vi "reward_behavior_michelle_visjitter.vi"() -> ()   [LabVIEW 2019]
doc: "The myRIO Project template acquires acceleration data from the onboard accelerometer and displays the changes of acceleration values in a waveform chart."
uses:
  <vilib>/myRIO/Common/Instrument Driver Framework/Utilities/typedefs/Generic FPGA Reference.ctl
  <vilib>/myRIO/Common/Instrument Driver Framework/Utilities/typedefs/myRIO v1.0 Reference.ctl
  <vilib>/myRIO/Common/Instrument Driver Framework/Utilities/typedefs/Hardware Version Enum.ctl
  <vilib>/myRIO/Common/Instrument Driver Framework/Utilities/typedefs/myRIO Generic Hardware Reference.ctl
  <vilib>/userdefined/High Color/nirio_resource_hc.ctl
  <vilib>/myRIO/Common/Instrument Driver Framework/Utilities/vis/Is FPGA Ref Available.vi
  <vilib>/myRIO/Common/Instrument Driver Framework/myRIO v1.0/Encoder/typedefs/Encoder Signal Mode.ctl
  <vilib>/myRIO/Common/Instrument Driver Framework/myRIO v1.0/Encoder/typedefs/Encoder Channels Enum.ctl
  <vilib>/myRIO/Instrument Drivers/Onboard IO/Encoder/typedefs/Encoder Reference.ctl
  <vilib>/myRIO/Instrument Drivers/Onboard IO/Encoder/Encoder.lvlib
  <vilib>/myRIO/Instrument Drivers/Onboard IO/Encoder/vis/Read.vi
  <vilib>/myRIO/Common/Instrument Driver Framework/myRIO v1.0/Encoder/typedefs/Encoder Configuration v1.0.ctl
  <vilib>/myRIO/Common/Instrument Driver Framework/myRIO v1.0/Encoder/vis/myRIO v1.1 Open Encoder.vi
  <vilib>/myRIO/Common/Instrument Driver Framework/myRIO v1.0/Encoder/vis/myRIO v1.0 Configure Encoder.vi
  <vilib>/myRIO/Instrument Drivers/Onboard IO/Encoder/vis/myRIO Encoder Open.xnode
  <vilib>/myRIO/Express VI/Onboard IO/Encoder/Encoder Express VI.xnode
  <vilib>/myRIO/Express VI/Onboard IO/DI/DI Express VI.xnode
  <vilib>/myRIO/Instrument Drivers/Onboard IO/DIO/vis/Read.vi
  <vilib>/myRIO/Instrument Drivers/Onboard IO/DIO/DIO.lvlib
  <vilib>/myRIO/Common/Instrument Driver Framework/myRIO v1.0/DIO/typedefs/DIO Channels Enum.ctl
  <vilib>/myRIO/Common/Instrument Driver Framework/myRIO v1.0/DIO/typedefs/DIO Channels List.ctl
  <vilib>/myRIO/Instrument Drivers/Onboard IO/DIO/typedefs/DIO Reference.ctl
  <vilib>/myRIO/Instrument Drivers/Onboard IO/DIO/vis/myRIO DIO Open.xnode
  <vilib>/myRIO/Common/Instrument Driver Framework/myRIO v1.0/DIO/vis/myRIO v1.1 Open DIO.vi
  <vilib>/myRIO/Instrument Drivers/Onboard IO/DIO/vis/Write.vi
  <vilib>/myRIO/Express VI/Onboard IO/DO/DO Express VI.xnode
  <vilib>/Analysis/Matrix/Datatypes/RealMatrix.ctl
  <vilib>/Analysis/Matrix/NI_Matrix.lvlib
panel:
  in  "Give reward":bool
  out "Timings":dbl[](array[numeric])
  out "ISI":dbl
  out "ISI start time":dbl
  out "Time_out":bool=TRUE
  out "Time since lick":dbl
  out "Time of last lick":dbl
  out "Rewarded trials":dbl[](array[numeric])
  out "Rewards":u16
  out "Active Trial":bool
  out "Array temp2":T1
  out "Stimuli Loaded":bool
  out "Stim_ID":dbl[](array[numeric])
  out "Reward_mat":dbl[](array[numeric])
  out "Reward":bool=TRUE
  out "Frame clock":i32
  out "Licks":u32
  out "Lick":bool
  out "Time":dbl
  out "Stop":bool
  in  "Frames to collect":u32
  out "Overflow?":bool
  out "Counter Value":i32
  out "Velocity":dbl
  out "Velocity Plot":dbl[](graph)
  out "Velocity array":dbl[](array[numeric])
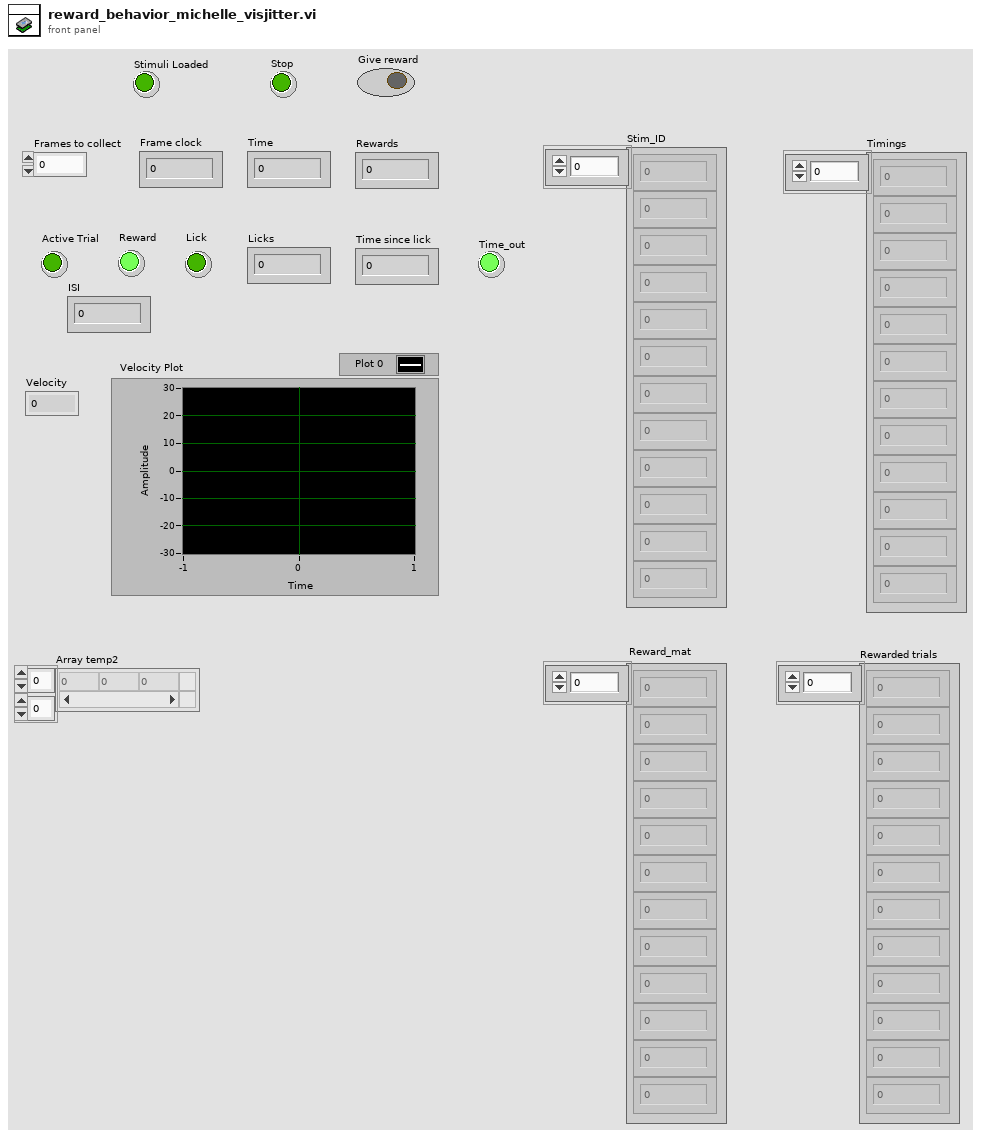
[diagram p1: front panel]
types:
  T1 = typedef "NI_Matrix.lvlib/RealMatrix.ctl" = dbl[][]
  T2 = typedef "Encoder.lvlib/Encoder Reference.ctl" = cluster{"myRIO Reference":T3, "Encoder Channels Enum":T7}
  T3 = typedef "myRIO Generic Hardware Reference.ctl" = cluster{"myRIO Model":T4, "myRIO Hardware Reference":T5}
  T4 = typedef "Hardware Version Enum.ctl" = enum16{"Unknown", "myRIO-1900", "myRIO-1950", "roboRIO", "NI ELVIS RIO CM", "ELVIS III"}
  T5 = typedef "myRIO v1.0 Reference.ctl" = cluster{"Generic FPGA Reference":T6, "Allow multiple opens":bool}
  T6 = typedef "Generic FPGA Reference.ctl" = refnum<k20>
  T7 = typedef "Encoder Channels Enum.ctl" = enum16{"Not Connected", "C/ENC0", "C/ENC1", "A/ENC", "A/ENC0", "A/ENC1", "A/ENC2", "A/ENC3", "A/ENC4", "A/ENC5", "A/ENC6", "A/ENC7", "A/ENC8", "A/ENC9", "B/ENC", "B/ENC0", "B/ENC1", "B/ENC2", "B/ENC3", "B/ENC4", "B/ENC5", "B/ENC6", "B/ENC7", "B/ENC8", "B/ENC9", "DIO/ENC0", "DIO/ENC1", "DIO/ENC2", "DIO/ENC3", "DIO/ENC4"}
  T8 = typedef "Encoder Signal Mode.ctl" = enum16{"Quadrature phase signal", "Step and direction signal"}
  T9 = typedef "nirio_resource_hc.ctl" = tag
  T10 = typedef "DIO.lvlib/DIO Reference.ctl" = cluster{"myRIO Reference":T3, "DIO Channels List":T11}
  T11 = typedef "DIO Channels List.ctl" = T12[]
  T12 = typedef "DIO Channels Enum.ctl" = enum16{"Not Connected", "C/DIO0", "C/DIO1", "C/DIO2", "C/DIO3", "C/DIO4", "C/DIO5", "C/DIO6", "C/DIO7", "A/DIO0", "A/DIO1", "A/DIO2", "A/DIO3", "A/DIO4", "A/DIO5", "A/DIO6", "A/DIO7", "A/DIO8", "A/DIO9", "A/DIO10", "A/DIO11", "A/DIO12", "A/DIO13", "A/DIO14", "A/DIO15", "A/DIO16", "A/DIO17", "A/DIO18", "A/DIO19", "B/DIO0", "B/DIO1", "B/DIO2", "B/DIO3", "B/DIO4", "B/DIO5", "B/DIO6", "B/DIO7", "B/DIO8", "B/DIO9", "B/DIO10", "B/DIO11", "B/DIO12", "B/DIO13", "B/DIO14", "B/DIO15", "B/DIO16", "B/DIO17", "B/DIO18", "B/DIO19", "LED0", "LED1", "LED2", "LED3", "Button0", "DIO/DIO0", "DIO/DIO1", "DIO/DIO2", "DIO/DIO3", "DIO/DIO4", "DIO/DIO5", "DIO/DIO6", "DIO/DIO7", "DIO/DIO8", "DIO/DIO9", "SPI/CS0", "SPI/CS1", "SPI/CS2", "SPI/CS3", "LED RADIO (Green)", "LED RADIO (Red)", "LED COMM (Green)", "LED COMM (Red)", "LED MODE (Green)", "LED MODE (Red)"}
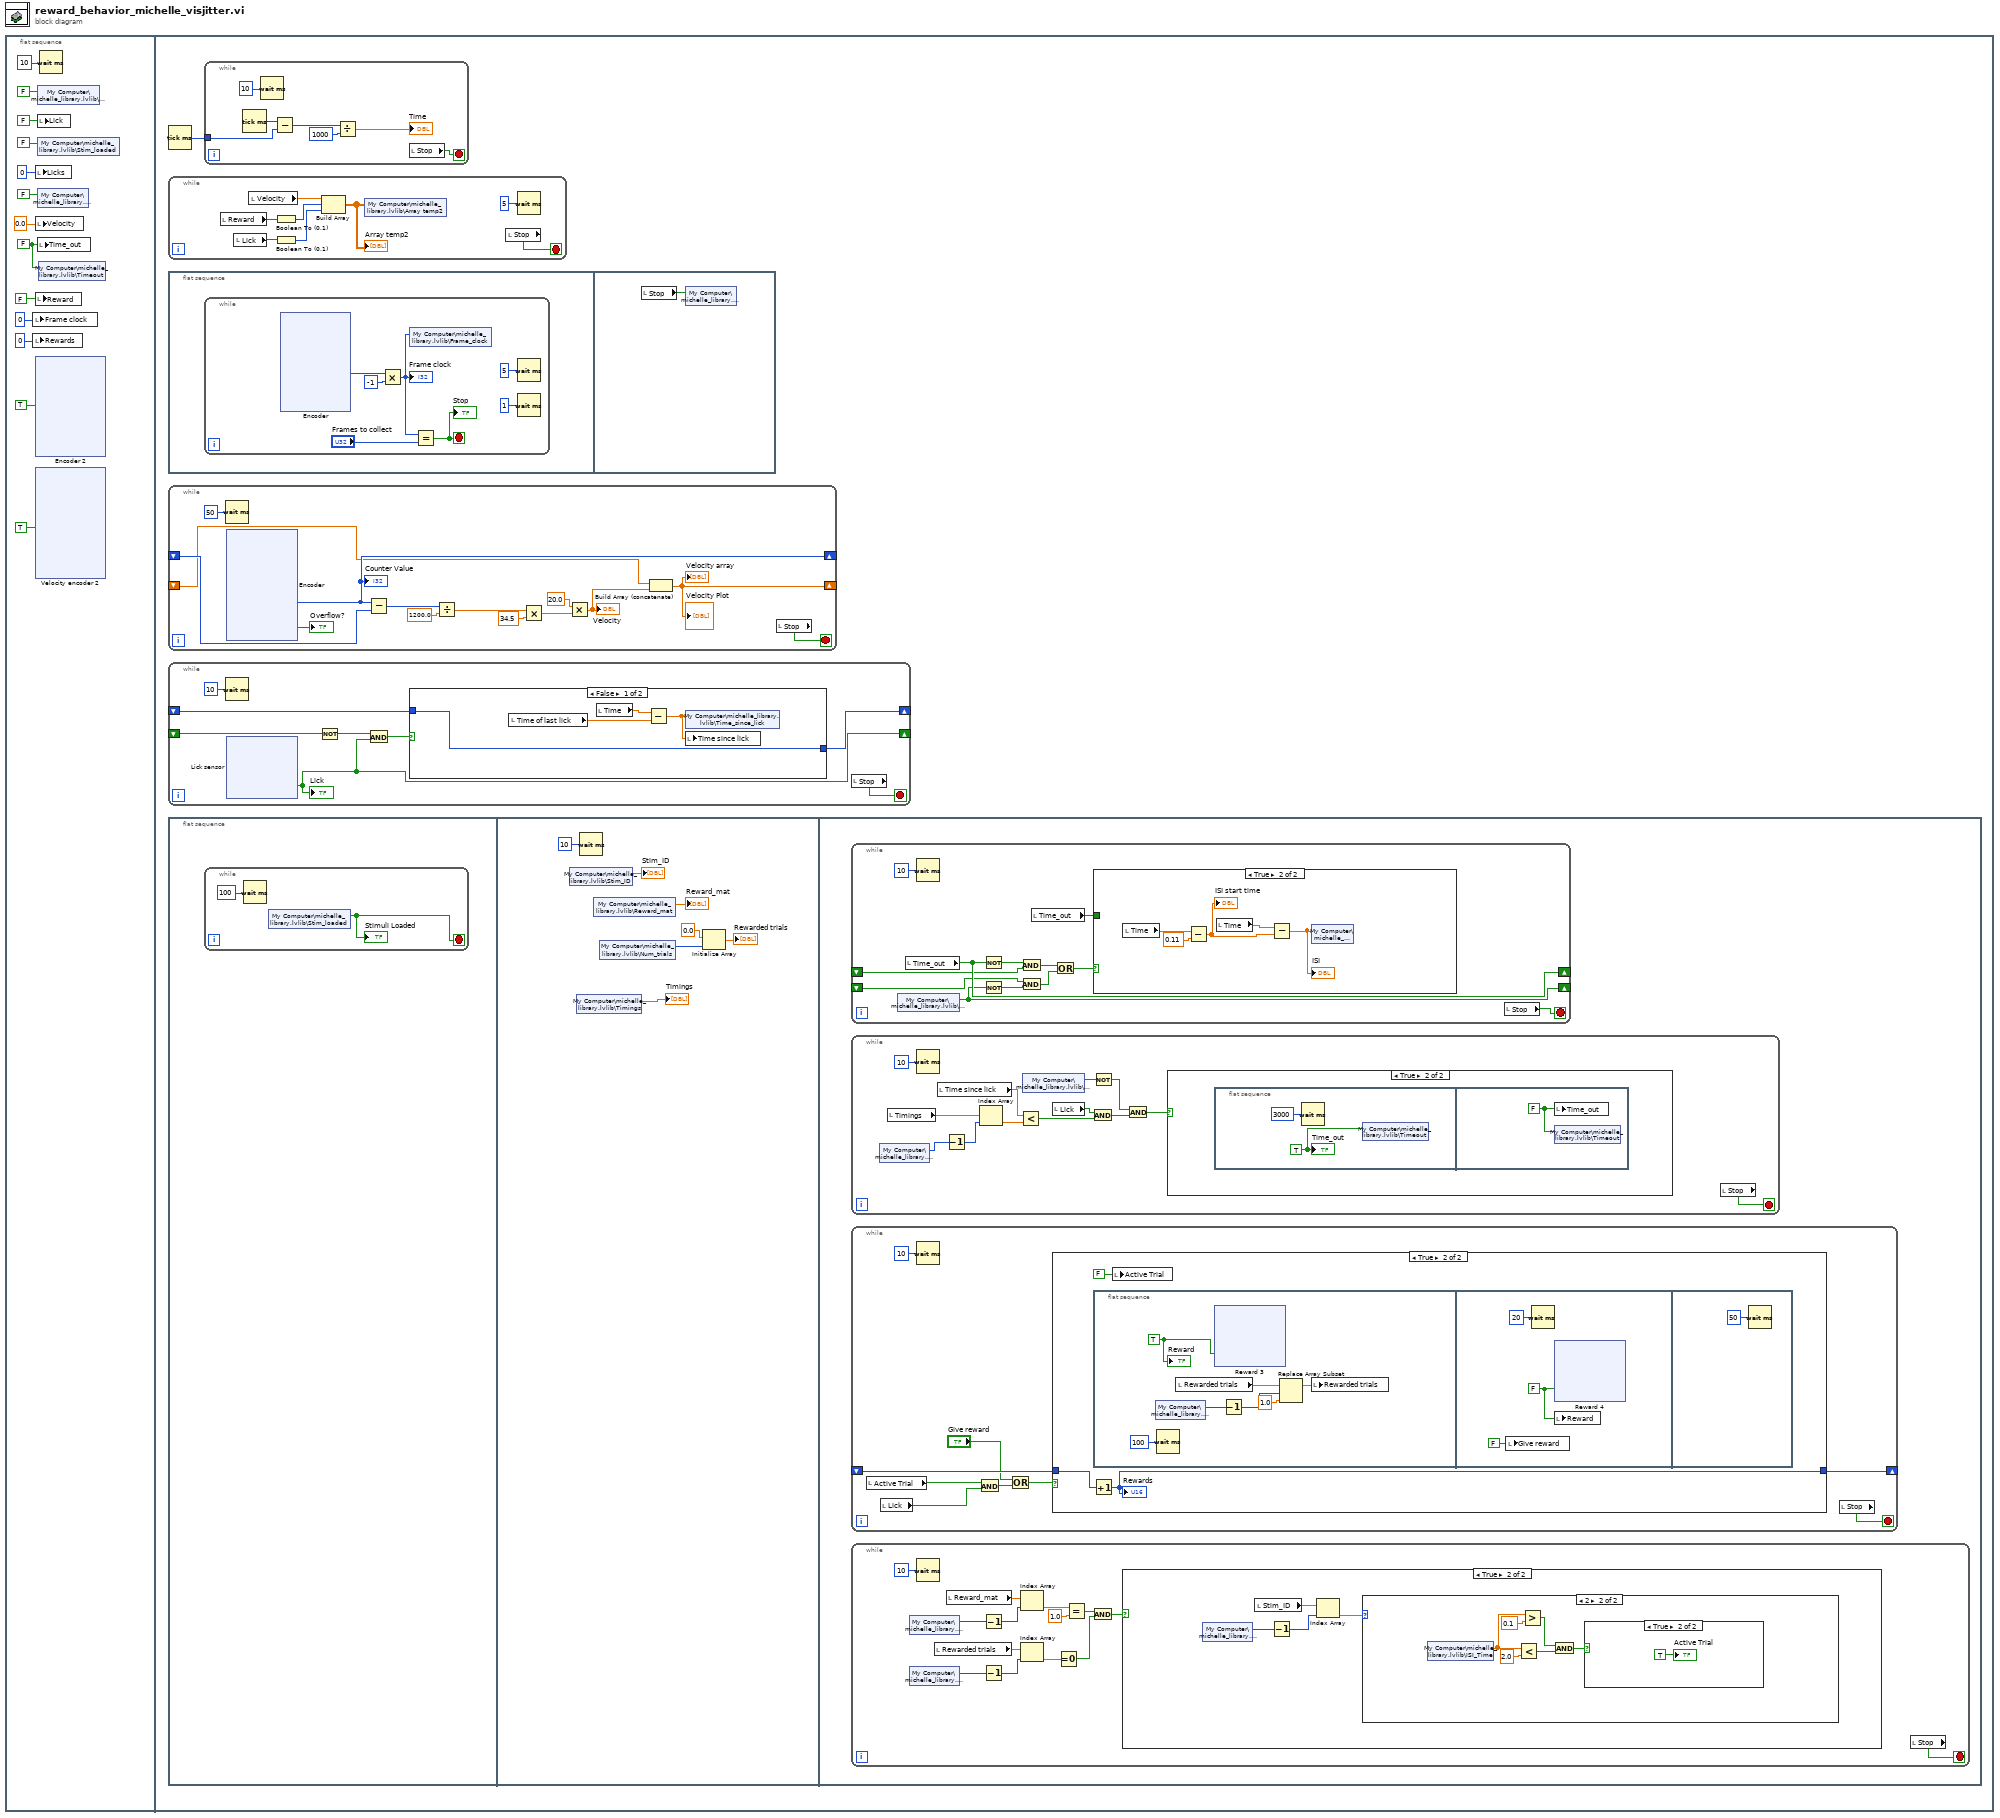
[diagram p0: block diagram]
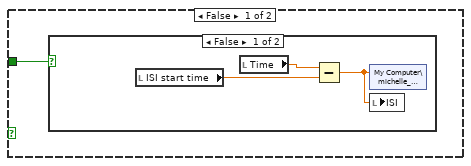
[diagram p3: hidden frame]
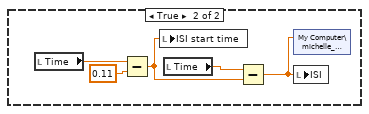
[diagram p4: hidden frame]
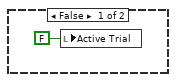
[diagram p5: hidden frame]
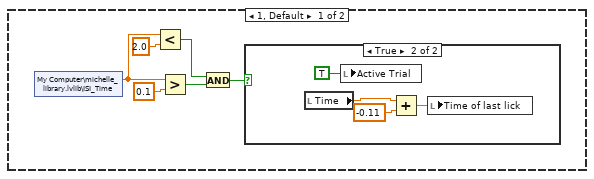
[diagram p6: hidden frame]
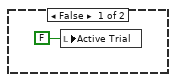
[diagram p7: hidden frame]
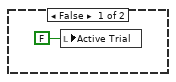
[diagram p8: hidden frame]
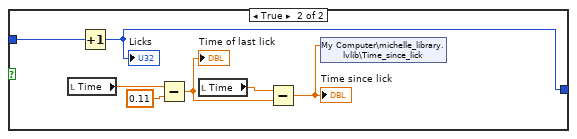
[diagram p10: hidden frame]
diagram:
  n1 = flat-sequence {
    frame #0 {
      w1 = FALSE ("Time_out")
      n2 = local write "Frame clock"(u32 0 ("Frames")) -> ()
      n3 = local write "Rewards"(u16 0 ("Rewards")) -> ()
      n4 = local write "Licks"(u32 0 ("Licks")) -> ()
      n5 = local write "Velocity"(0.0 ("Velocity")) -> ()
      n6 = local write "Reward"(FALSE ("Give reward")) -> ()
      n7 = xnode "Encoder 2"("Reset Counter"=TRUE) -> ()  [unwired: 1 in, 4 out]
      n8 = xnode "Velocity encoder 2"("Reset Counter"=TRUE) -> ()  [unwired: 1 in, 4 out]
      n9 = shared-variable "My Computer\\michelle_library.lvlib\\Display"(FALSE ("Display")) -> ()  [unwired: 1 in, 1 out]
      n10 = local write "Lick"(FALSE ("Lick")) -> ()
      n11 = shared-variable "My Computer\\michelle_library.lvlib\\Stim_loaded"(FALSE ("Stim_loaded")) -> ()  [unwired: 1 in, 1 out]
      n12 = shared-variable "My Computer\\michelle_library.lvlib\\Stop"(FALSE ("Stop")) -> ()  [unwired: 1 in, 1 out]
      n13 = local write "Time_out"(w1) -> ()
      n14 = shared-variable "My Computer\\michelle_library.lvlib\\Timeout"(w1) -> ()  [unwired: 1 in, 1 out]
      n15 = Wait (ms)(milliseconds to wait=u32 10) -> ()  [unwired: 1 out]
    }
    frame #1 {
      n16 = Tick Count (ms)() -> (millisecond timer value=w106:u32)
      n17 = while {
        stop <- w108 stop-if-true
        n18 = local read "Reward"() -> (w113:bool)
        n19 = local read "Lick"() -> (w114:bool)
        n20 = local read "Velocity"() -> (w112:dbl)
        n21 = Boolean To (0,1)(Boolean=w113) -> (0, 1=w111:i16)
        n22 = Boolean To (0,1)(Boolean=w114) -> (0, 1=w110:i16)
        n23 = Build Array(w112, w111, w110) -> (w107:T1)
        "Array temp2" <- w107
        n24 = shared-variable "My Computer\\michelle_library.lvlib\\Array temp2"(w107) -> ()  [unwired: 1 in, 1 out]
        n25 = local read "Stop"() -> (w108:bool)
        n26 = Wait (ms)(milliseconds to wait=u32 5) -> ()  [unwired: 1 out]
      }
      n27 = flat-sequence {
        frame #0 {
          n28 = while {
            stop <- w299 stop-if-true
            n29 = xnode "Encoder"() -> ("Counter Value"=w303:i32)  [unwired: 2 in, 3 out]
            n30 = Multiply(x=w303, y=-1) -> (x*y=w298:i32)
            "Frame clock" <- w298
            n31 = shared-variable "My Computer\\michelle_library.lvlib\\Frame_clock"(w298) -> ()  [unwired: 1 in, 1 out]
            n32 = Equal?(x=w298, y="Frames to collect") -> (x = y?=w299:bool)
            "Stop" <- w299
            n33 = Wait (ms)(milliseconds to wait=u32 5) -> ()  [unwired: 1 out]
            n34 = Wait (ms)(milliseconds to wait=u32 1) -> ()  [unwired: 1 out]
          }
        }
        frame #1 {
          n35 = local read "Stop"() -> (w351:bool)
          n36 = shared-variable "My Computer\\michelle_library.lvlib\\Stop"(w351) -> ()  [unwired: 1 in, 1 out]
        }
      }
      n37 = while {
        shift-right: [w416] -> _
        shift-left: _ -> [w417]
        shift-right: [w408] -> _
        shift-left: _ -> [w407]
        stop <- w406 stop-if-true
        n38 = Wait (ms)(milliseconds to wait=u32 50) -> ()  [unwired: 1 out]
        n39 = xnode "Encoder"() -> ("Counter Value"=w416:i32, "Overflow?"=→"Overflow?":bool)  [unwired: 2 in, 2 out]
        "Counter Value" <- w416
        n40 = Subtract(x=w416, y=w417) -> (x-y=w409:i32)
        n41 = Divide(x=w409, y=1200.0 ("600")) -> (x/y=w414:dbl)
        n42 = Multiply(x=w414, y=34.5) -> (x*y=w412:dbl)
        n43 = Multiply(x=20.0, y=w412) -> (x*y=w410:dbl)
        "Velocity" <- w410
        n44 = Build Array (concatenate)(w407, w410) -> (w408:dbl[])
        "Velocity Plot" <- w408
        "Velocity array" <- w408
        n45 = local read "Stop"() -> (w406:bool)
      }
      n46 = while {
        shift-right: [w358] -> _
        shift-left: _ -> [w357]
        shift-right: [w352] -> _
        shift-left: _ -> [w355]
        stop <- w356 stop-if-true
        n47 = Wait (ms)(milliseconds to wait=u32 10) -> ()  [unwired: 1 out]
        n48 = xnode "Lick sensor"() -> ("C/DIO1 (DIO1)"=w352:bool)  [unwired: 1 in, 1 out]
        "Lick" <- w352
        n49 = Not(x=w355) -> (.not. x?=w354:bool)
        n50 = And(x=w354, y=w352) -> (x .and. y?=w353:bool)
        n51 = case shown="False" w353 {
          tunnel: [w363 w370] -> w358
          tunnel: w357 -> [w363 w369]
          frame False {
            n52 = local read "Time of last lick"() -> (w361:dbl)
            n53 = local read "Time"() -> (w362:dbl)
            n54 = Subtract(x=w362, y=w361) -> (x-y=w360:dbl)
            n55 = shared-variable "My Computer\\michelle_library.lvlib\\Time_since_lick"(w360) -> ()  [unwired: 1 in, 1 out]
            n56 = local write "Time since lick"(w360) -> ()
          }
          frame True {
            n57 = local read "Time"() -> (w366:dbl)
            n58 = Increment(x=w369) -> (x+1=w370:u32)
            "Licks" <- w370
            n59 = Subtract(x=w366, y=0.11) -> (x-y=w364:dbl)
            "Time of last lick" <- w364
            n60 = local read "Time"() -> (w368:dbl)
            n61 = Subtract(x=w368, y=w364) -> (x-y=w367:dbl)
            "Time since lick" <- w367
            n62 = shared-variable "My Computer\\michelle_library.lvlib\\Time_since_lick"(w367) -> ()  [unwired: 1 in, 1 out]
          }
        }
        n63 = local read "Stop"() -> (w356:bool)
      }
      n64 = flat-sequence {
        frame #0 {
          n65 = while {
            stop <- w116 stop-if-true
            n66 = Wait (ms)(milliseconds to wait=u32 100) -> ()  [unwired: 1 out]
            n67 = shared-variable "My Computer\\michelle_library.lvlib\\Stim_loaded"() -> (w116:bool)  [unwired: 1 in, 1 out]
            "Stimuli Loaded" <- w116
          }
        }
        frame #1 {
          n68 = shared-variable "My Computer\\michelle_library.lvlib\\Stim_ID"() -> (→"Stim_ID":dbl[])  [unwired: 1 in, 1 out]
          n69 = shared-variable "My Computer\\michelle_library.lvlib\\Timings"() -> (→"Timings":dbl[])  [unwired: 1 in, 1 out]
          n70 = Wait (ms)(milliseconds to wait=u32 10) -> ()  [unwired: 1 out]
          n71 = shared-variable "My Computer\\michelle_library.lvlib\\Reward_mat"() -> (→"Reward_mat":dbl[])  [unwired: 1 in, 1 out]
          n72 = shared-variable "My Computer\\michelle_library.lvlib\\Num_trials"() -> (w120:u32)  [unwired: 1 in, 1 out]
          n73 = Initialize Array(0.0 ("element"), w120) -> (→"Rewarded trials":dbl[])
        }
        frame #2 {
          n74 = while {
            shift-right: [w150] -> _
            shift-left: _ -> [w148]
            shift-right: [w146] -> _
            shift-left: _ -> [w145]
            stop <- w151 stop-if-true
            n75 = shared-variable "My Computer\\michelle_library.lvlib\\Display"() -> (w146:bool)  [unwired: 1 in, 1 out]
            n76 = local read "Time_out"() -> (w150:bool)
            n77 = Wait (ms)(milliseconds to wait=u32 10) -> ()  [unwired: 1 out]
            n78 = Not(x=w150) -> (.not. x?=w149:bool)
            n79 = Not(x=w146) -> (.not. x?=w144:bool)
            n80 = And(x=w149, y=w148) -> (x .and. y?=w143:bool)
            n81 = And(x=w145, y=w144) -> (x .and. y?=w142:bool)
            n82 = local read "Time_out"() -> (w147:bool)
            n83 = Or(x=w143, y=w142) -> (x .or. y?=w141:bool)
            n84 = case shown="True" w141 {
              tunnel: w147 -> [w152 _]
              frame False {
                n85 = case shown="False" w152 {
                  frame False {
                    n86 = local read "ISI start time"() -> (w155:dbl)
                    n87 = local read "Time"() -> (w154:dbl)
                    n88 = Subtract(x=w154, y=w155) -> (x-y=w153:dbl)
                    n89 = shared-variable "My Computer\\michelle_library.lvlib\\ISI"(w153) -> ()  [unwired: 1 in, 1 out]
                    n90 = local write "ISI"(w153) -> ()
                  }
                  frame True {
                    n91 = local read "Time"() -> (w160:dbl)
                    n92 = Subtract(x=w160, y=0.11) -> (x-y=w157:dbl)
                    n93 = local write "ISI start time"(w157) -> ()
                    n94 = local read "Time"() -> (w158:dbl)
                    n95 = Subtract(x=w158, y=w157) -> (x-y=w156:dbl)
                    n96 = shared-variable "My Computer\\michelle_library.lvlib\\ISI"(w156) -> ()  [unwired: 1 in, 1 out]
                    n97 = local write "ISI"(w156) -> ()
                  }
                }
              }
              frame True {
                n98 = local read "Time"() -> (w165:dbl)
                n99 = Subtract(x=w165, y=0.11) -> (x-y=w162:dbl)
                "ISI start time" <- w162
                n100 = local read "Time"() -> (w163:dbl)
                n101 = Subtract(x=w163, y=w162) -> (x-y=w161:dbl)
                "ISI" <- w161
                n102 = shared-variable "My Computer\\michelle_library.lvlib\\ISI"(w161) -> ()  [unwired: 1 in, 1 out]
              }
            }
            n103 = local read "Stop"() -> (w151:bool)
          }
          n104 = while {
            stop <- w136 stop-if-true
            n105 = shared-variable "My Computer\\michelle_library.lvlib\\Trial"() -> (w125:u32)  [unwired: 1 in, 1 out]
            n106 = local read "Timings"() -> (w127:dbl[])
            n107 = Wait (ms)(milliseconds to wait=u32 10) -> ()  [unwired: 1 out]
            n108 = local read "Time since lick"() -> (w135:dbl)
            n109 = Decrement(x=w125) -> (x-1=w124:u32)
            n110 = Index Array(array=w127, index=w124) -> (element=w126:dbl)
            n111 = Less?(x=w135, y=w126) -> (x < y?=w134:bool)
            n112 = shared-variable "My Computer\\michelle_library.lvlib\\Display"() -> (w131:bool)  [unwired: 1 in, 1 out]
            n113 = local read "Lick"() -> (w133:bool)
            n114 = Not(x=w131) -> (.not. x?=w130:bool)
            n115 = And(x=w133, y=w134) -> (x .and. y?=w129:bool)
            n116 = And(x=w130, y=w129) -> (x .and. y?=w128:bool)
            n117 = case shown="True" w128 {
              frame False {
              }
              frame True {
                n118 = flat-sequence {
                  frame #0 {
                    w138 = TRUE
                    n119 = Wait (ms)(milliseconds to wait=u32 3000) -> ()  [unwired: 1 out]
                    n120 = shared-variable "My Computer\\michelle_library.lvlib\\Timeout"(w138) -> ()  [unwired: 1 in, 1 out]
                    "Time_out" <- w138
                  }
                  frame #1 {
                    w139 = FALSE ("Timeout")
                    n121 = local write "Time_out"(w139) -> ()
                    n122 = shared-variable "My Computer\\michelle_library.lvlib\\Timeout"(w139) -> ()  [unwired: 1 in, 1 out]
                  }
                }
              }
            }
            n123 = local read "Stop"() -> (w136:bool)
          }
          n124 = while {
            shift-right: [w210] -> _
            shift-left: _ -> [w209]
            stop <- w212 stop-if-true
            n125 = local read "Active Trial"() -> (w207:bool)
            n126 = local read "Lick"() -> (w208:bool)
            n127 = Wait (ms)(milliseconds to wait=u32 10) -> ()  [unwired: 1 out]
            n128 = And(x=w207, y=w208) -> (x .and. y?=w206:bool)
            n129 = Or(x="Give reward", y=w206) -> (x .or. y?=w205:bool)
            n130 = case shown="True" w205 {
              tunnel: [w213 w216] -> w210
              tunnel: w209 -> [w213 w215]
              frame False {
              }
              frame True {
                n131 = Increment(x=w215) -> (x+1=w216:u16)
                "Rewards" <- w216
                n132 = flat-sequence {
                  frame #0 {
                    w222 = TRUE ("C/DIO0 (DIO0)")
                    n133 = shared-variable "My Computer\\michelle_library.lvlib\\Trial"() -> (w221:u32)  [unwired: 1 in, 1 out]
                    n134 = Wait (ms)(milliseconds to wait=u32 100) -> ()  [unwired: 1 out]
                    n135 = local read "Rewarded trials"() -> (w219:dbl[])
                    n136 = xnode "Reward 3"("C/DIO0 (DIO0)"=w222) -> ()  [unwired: 1 in, 1 out]
                    n137 = Decrement(x=w221) -> (x-1=w220:u32)
                    n138 = Replace Array Subset(array=w219, new element=1.0 ("new element/subarray"), index=w220) -> (w217:dbl[])
                    n139 = local write "Rewarded trials"(w217) -> ()
                    "Reward" <- w222
                  }
                  frame #1 {
                    w261 = FALSE ("C/DIO0 (DIO0)")
                    n140 = local write "Give reward"(FALSE ("Give reward")) -> ()
                    n141 = Wait (ms)(milliseconds to wait=u32 20) -> ()  [unwired: 1 out]
                    n142 = xnode "Reward 4"("C/DIO0 (DIO0)"=w261) -> ()  [unwired: 1 in, 1 out]
                    n143 = local write "Reward"(w261) -> ()
                  }
                  frame #2 {
                    n144 = Wait (ms)(milliseconds to wait=u32 50) -> ()  [unwired: 1 out]
                  }
                }
                n145 = local write "Active Trial"(FALSE ("Active Trial")) -> ()
              }
            }
            n146 = local read "Stop"() -> (w212:bool)
          }
          n147 = while {
            stop <- w179 stop-if-true
            n148 = shared-variable "My Computer\\michelle_library.lvlib\\Trial"() -> (w175:u32)  [unwired: 1 in, 1 out]
            n149 = shared-variable "My Computer\\michelle_library.lvlib\\Trial"() -> (w171:u32)  [unwired: 1 in, 1 out]
            n150 = Wait (ms)(milliseconds to wait=u32 10) -> ()  [unwired: 1 out]
            n151 = local read "Rewarded trials"() -> (w172:dbl[])
            n152 = local read "Reward_mat"() -> (w174:dbl[])
            n153 = Decrement(x=w175) -> (x-1=w176:u32)
            n154 = Decrement(x=w171) -> (x-1=w170:u32)
            n155 = Index Array(array=w174, index=w176) -> (element=w177:dbl)
            n156 = Index Array(array=w172, index=w170) -> (element=w169:dbl)
            n157 = Equal To 0?(x=w169) -> (x = 0?=w168:bool)
            n158 = Equal?(x=w177, y=1.0) -> (x = y?=w167:bool)
            n159 = And(x=w167, y=w168) -> (x .and. y?=w166:bool)
            n160 = case shown="True" w166 {
              frame False {
                n161 = local write "Active Trial"(FALSE ("Active_trial")) -> ()
              }
              frame True {
                n162 = shared-variable "My Computer\\michelle_library.lvlib\\Trial"() -> (w182:u32)  [unwired: 1 in, 1 out]
                n163 = local read "Stim_ID"() -> (w184:dbl[])
                n164 = Decrement(x=w182) -> (x-1=w183:u32)
                n165 = Index Array(array=w184, index=w183) -> (element=w181:dbl)
                n166 = case shown="2" w181 {
                  frame 1, Default {
                    n167 = shared-variable "My Computer\\michelle_library.lvlib\\ISI_Time"() -> (w189:dbl)  [unwired: 1 in, 1 out]
                    n168 = Less?(x=w189, y=2.0) -> (x < y?=w187:bool)
                    n169 = Greater?(x=w189, y=0.1) -> (0:w186:bool)
                    n170 = And(x=w187, y=w186) -> (x .and. y?=w185:bool)
                    n171 = case shown="True" w185 {
                      frame False {
                        n172 = local write "Active Trial"(FALSE ("Active Trial")) -> ()
                      }
                      frame True {
                        n173 = local read "Time"() -> (w194:dbl)
                        n174 = local write "Active Trial"(TRUE ("Active Trial")) -> ()
                        n175 = Add(x=w194, y=-0.11) -> (x+y=w192:dbl)
                        n176 = local write "Time of last lick"(w192) -> ()
                      }
                    }
                  }
                  frame 2 {
                    n177 = shared-variable "My Computer\\michelle_library.lvlib\\ISI_Time"() -> (w200:dbl)  [unwired: 1 in, 1 out]
                    n178 = Less?(x=w200, y=2.0) -> (x < y?=w197:bool)
                    n179 = Greater?(x=w200, y=0.1) -> (0:w198:bool)
                    n180 = And(x=w198, y=w197) -> (x .and. y?=w196:bool)
                    n181 = case shown="True" w196 {
                      frame False {
                        n182 = local write "Active Trial"(FALSE ("Active Trial")) -> ()
                      }
                      frame True {
                        "Active Trial" <- TRUE ("Active Trial")
                      }
                    }
                  }
                }
              }
            }
            n183 = local read "Stop"() -> (w179:bool)
          }
        }
      }
      n184 = while {
        tunnel: w106 -> [w471]
        stop <- w469 stop-if-true
        n185 = Tick Count (ms)() -> (millisecond timer value=w472:u32)
        n186 = Wait (ms)(milliseconds to wait=u32 10) -> ()  [unwired: 1 out]
        n187 = Subtract(x=w472, y=w471) -> (x-y=w468:u32)
        n188 = Divide(x=w468, y=u32 1000) -> (x/y=→"Time":dbl)
        n189 = local read "Stop"() -> (w469:bool)
      }
    }
  }
